vi "OOB to Logic FGV.vi"(7 "Op (Get)":enum16{"Get", "Set"}(ring), 8 "error in (no error)":errorcluster, 11 "OOB to Logic Data in":T1) -> (0 "error out":errorcluster, 3 "OOB to Logic Data out":T1)   [LabVIEW 2025, in "OOB Data Transfer.lvlib"]
uses:
  OOB Data Transfer.lvlib
  Typdefs/OOB to Logic Data.ctl
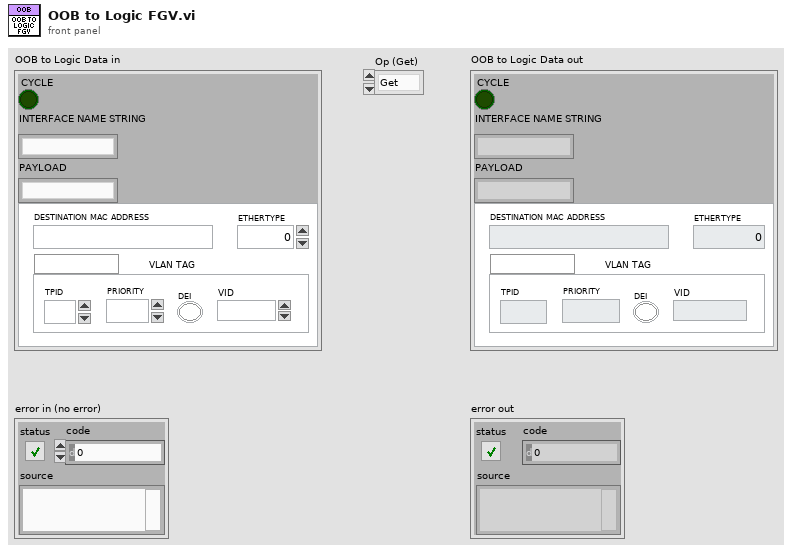
[diagram p1: front panel]
types:
  T1 = typedef "OOB Data Transfer.lvlib/OOB to Logic Data.ctl" = cluster{"CYCLE":bool, "INTERFACE NAME STRING":string, "PAYLOAD":string, "Protocol Layer":cluster{"Has VLAN":bool, "VLAN TAG":cluster{"TPID":u16, "PRIORITY":u8, "DEI":bool, "VID":u16}, "DESTINATION MAC ADDRESS":string, "ETHERTYPE":u16}}
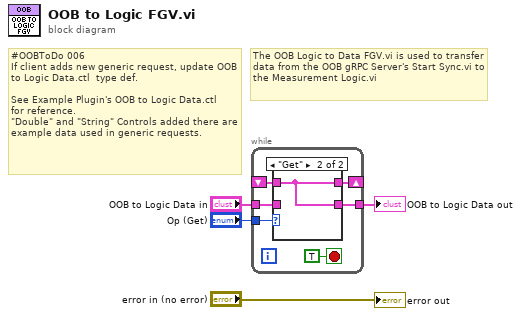
[diagram p0: block diagram]
diagram:
  # "The OOB Logic to Data FGV.vi is used to transfer data from the OOB gRPC Server's Start Sync.vi to the Measurement Logic.vi"
  # "#OOBToDo 006 \nIf client adds new generic request, update OOB to Logic Data.ctl  type def.\n \nSee Example Plugin's OOB to Logic Data.ctl for reference. \n\"Double\" and \"String\" Controls added there are example data used in generic requests."
  n1 = while {
    tunnel: "Op (Get)" -> [w9]
    tunnel: "OOB to Logic Data in" -> [w8]
    shift-right: [w7] -> _
    shift-left: _ -> [w6]
    tunnel: [w5] -> w1
    stop <- TRUE stop-if-true
    n2 = case shown="\"Get\"" w9 {
      tunnel: w8 -> [w11 _]
      tunnel: [w11 w12] -> w7
      tunnel: [w11 w12] -> w5
      tunnel: w6 -> [_ w12]
      frame "Set" {
      }
      frame "Get" {
      }
    }
  }
  "OOB to Logic Data out" <- w1
  "error out" <- "error in (no error)"
